vi "terminate.vi"(8 "error in (no error)":errorcluster, 11 "GenericPlugin in":refnum<class "LightSourceMH110125Tsunami.lvclass">) -> (0 "error out":errorcluster, 3 "GenericPlugin out":refnum<class "LightSourceMH110125Tsunami.lvclass">)   [LabVIEW 2010, in "LightSourceMH110125Tsunami.lvclass"]
doc: "The dynamic dispatch version of this VI terminates the plug-in object by releasing all of its resources."
uses:
  LightSourceMH110125Tsunami.lvclass
  LightSourceScaffold/LightSourceScaffold/LightSourceScaffold.lvclass
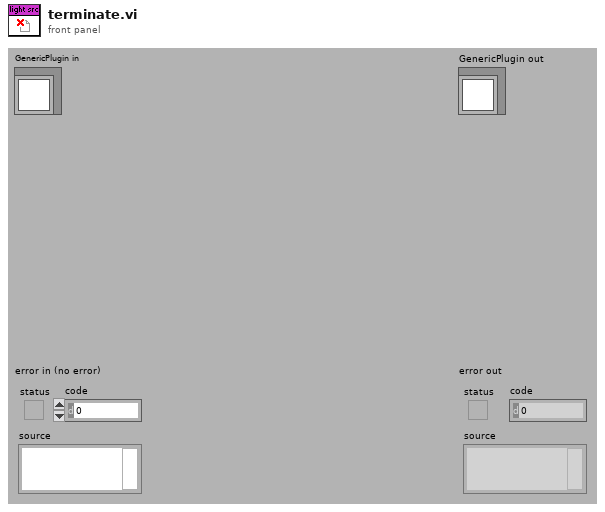
[diagram p1: front panel]
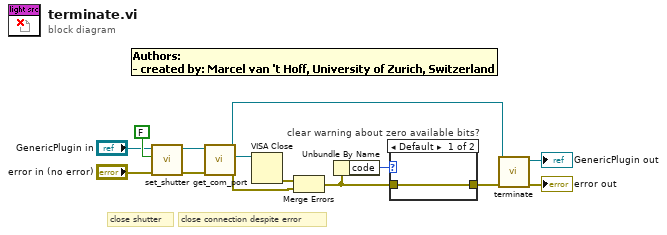
[diagram p0: block diagram]
diagram:
  # "close shutter"
  # "close connection despite error"
  n1 = call-dynamic "set_shutter.vi"("error in (no error)"="error in (no error)", "shutter open?"=FALSE, "LightSourceMH110125Tsunami in"="GenericPlugin in") -> ("error out"=w2:errorcluster, "LightSourceMH110125Tsunami out"=w5:refnum<class "LightSourceMH110125Tsunami.lvclass">)  [unwired: 6 in, 1 out]
  n2 = call-dynamic "get_com_port.vi"("error in (no error)"=w2, "LightSourceMH110125Tsunami in"=w5) -> ("error out"=w1:errorcluster, "comm port"=w3:refnum<visa-resource-name>, "LightSourceMH110125Tsunami out"=w4:refnum<class "LightSourceMH110125Tsunami.lvclass">)  [unwired: 7 in]
  n3 = VISA Close(VISA resource name=w3) -> (error out=w11:errorcluster)  [unwired: 1 in]
  n4 = Merge Errors(w11, w1) -> (w9:errorcluster)
  n5 = Unbundle By Name(w9) -> ("code"=w10:i32)
  n6 = case "clear warning about zero available bits?" shown="Default" w10 {
    tunnel: [w15 _] -> w6
    tunnel: w9 -> [w15 _]
    frame Default {
    }
    frame 1073676294 {
    }
  }
  n7 = call-parent "terminate.vi"("error in (no error)"=w6, "GenericPlugin in"=w4) -> ("error out"=→"error out":errorcluster, "GenericPlugin out"=→"GenericPlugin out":refnum<class "LightSourceMH110125Tsunami.lvclass">)  [unwired: 8 in]
